vi "ActionVIOnCompile.vi"(8 "error in":errorcluster, 11 "Device Item Ref in":T1 format="%.0x") -> (0 "error out":errorcluster)   [LabVIEW 2017, in "Waveform-Processing-Custom-Device System Explorer.lvlib"]
uses:
  Waveform-Processing-Custom-Device System Explorer.lvlib
  <vilib>/NI Veristand/Custom Device API/Custom Device Item Ref.ctl
  Shared/Types/FG Action.ctl
  Shared/CompiledSettings.ctl
  <vilib>/NI Veristand/Custom Device API/Block Data Reference.ctl
  <vilib>/NI Veristand/Custom Device API/Data Reference.ctl
  <vilib>/NI Veristand/Custom Device API/Waveform Data Reference.ctl
  Shared/Constants.vi
  <vilib>/NI Veristand/Custom Device API/Set Item Property (Variant).vi
  <vilib>/NI Veristand/Custom Device API/Custom Device API.lvlib
  <vilib>/NI/NIVS Inline Async API/_Data Access System Explorer/Data Access System Explorer.lvlib
  Shared/Waveform-Processing-Custom-Device Shared.lvlib
  Shared/Running Average/Running Average.lvlib
  Shared/Single Point/SinglePoint.lvlib
  Shared/Max Single Point/Max_SP.lvlib
  Shared/Min Single Point/Min_SP.lvlib
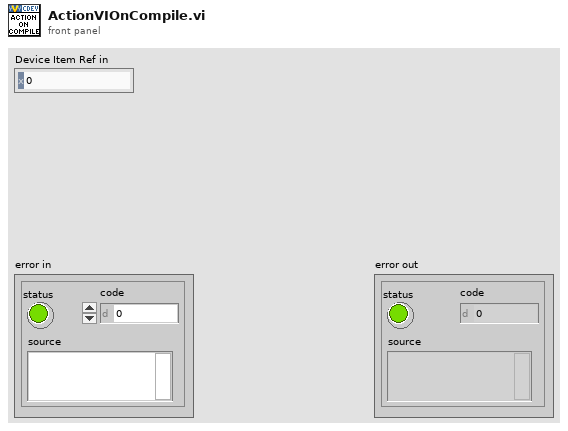
[diagram p1: front panel]
types:
  T1 = typedef "Custom Device API.lvlib/Custom Device Item Ref.ctl" = u64
  T2 = typedef "Waveform-Processing-Custom-Device Shared.lvlib/CompiledSettings.ctl" = cluster{"Name":string, "Buffer Length (samples)":u32, "Enable Array":bool[], "Parameter Block Data Refs":T3[], "Source Wfm Data Refs":T5[], "Result Wfm Data Refs":T5[], "Result Ch Data Refs":T4[], "Task Rate (Hz)":dbl}
  T3 = typedef "Custom Device API.lvlib/Block Data Reference.ctl" = cluster{"Data Reference":T4, "Offset":u64, "Length":u64}
  T4 = typedef "Custom Device API.lvlib/Data Reference.ctl" = i32
  T5 = typedef "Custom Device API.lvlib/Waveform Data Reference.ctl" = i32
  T6 = typedef "Waveform-Processing-Custom-Device Shared.lvlib/FG Action.ctl" = enum8{"GET", "SET"}
  T7 = typedef "Custom Device API.lvlib/Custom Device Item Info.ctl" = cluster{"Name":string, "Is Channel":bool, "GUID":string, "Is Waveform":bool}
  T8 = typedef "Waveform-Processing-Custom-Device Shared.lvlib/Custom Device Settings.ctl" = cluster{"CD Task Dependency":T1, "CD Task Dependency Ref":T1, "CD Task Available Wfms":string[], "CD Task Selected Wfms":string[], "Buffer Length (samples)":u32, "Min Enabled":bool, "Max Enabled ":bool, "SP Enabled":bool, "RMS Enabled":bool, "Buffer Length (s)":dbl, "Task Rate":dbl, "Number of DAQ Chanels":u32}
  T9 = cluster{"Name":string, "Type":enum16{"Output/Write", "Input/Read", "Input/ReadWrite"}, "VS Refs":T1[]}[]
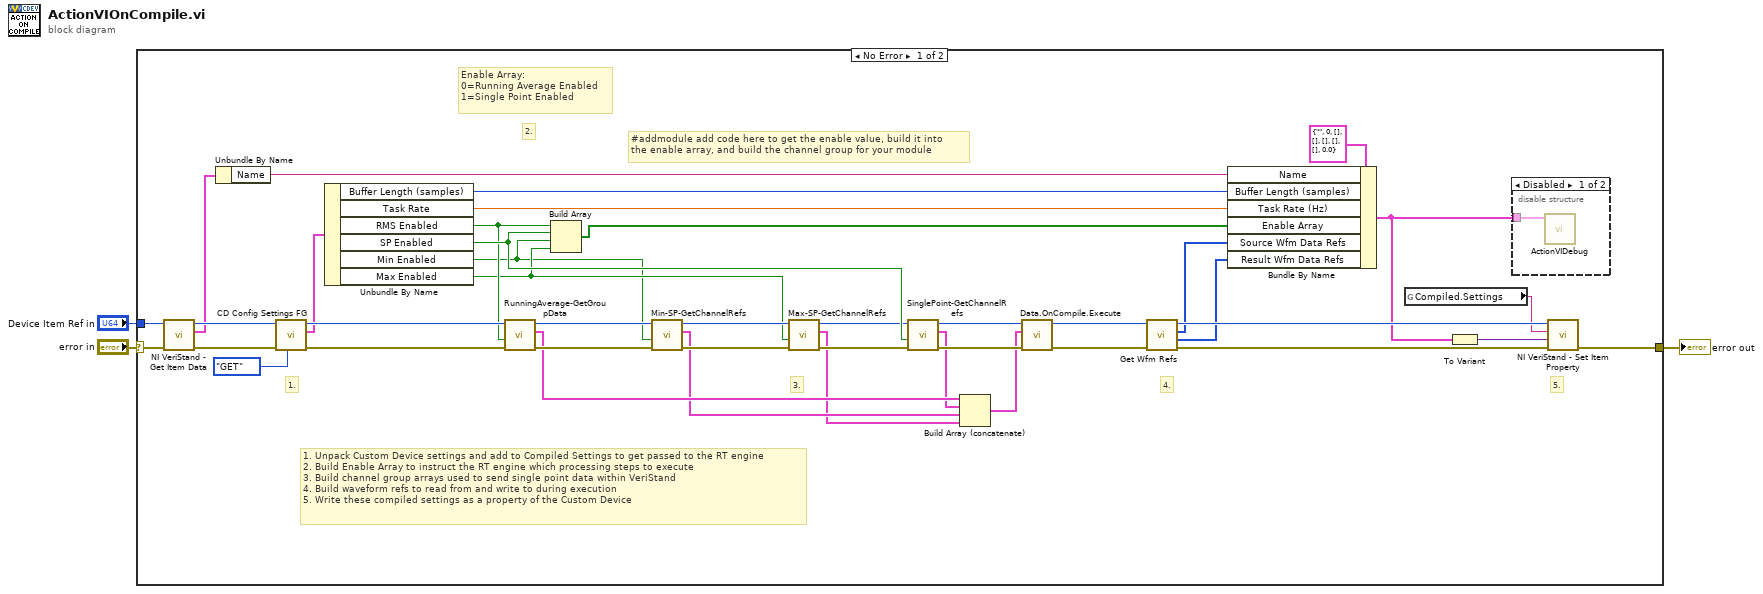
[diagram p0: block diagram]
diagram:
  n1 = case shown="No Error" "error in" {
    selector: "error in" -> [w43 w46]
    tunnel: [w44 w46] -> w2
    tunnel: "Device Item Ref in" -> [w42 _]
    frame No Error {
      # "#addmodule add code here to get the enable value, build it into\nthe enable array, and build the channel group for your module"
      # "Enable Array:\n0=Running Average Enabled\n1=Single Point Enabled"
      # "5."
      # "4."
      # "3."
      # "2."
      # "1."
      # "1. Unpack Custom Device settings and add to Compiled Settings to get passed to the RT engine\n2. Build Enable Array to instruct the RT engine which processing steps to execute\n3. Build channel group arrays used to send single point data within VeriStand\n4. Build waveform refs to read from and write to during execution\n5. Write these compiled settings as a property of the Custom Device"
      n2 = call <vilib>:"NI VeriStand - Get Item Data.vi"("error in (no error)"=w43, "Item Ref in"=w42) -> ("error out"=w40:errorcluster, "Item Info"=w39:T7, "Item Ref out"=w41:T1)  [unwired: 6 in, 1 out]
      n3 = Unbundle By Name(w39) -> ("Name"=w31:string)
      n4 = call "CD Config Settings FG.vi"("Action"=FG_Action."GET", "Error In"=w40, "Item Ref"=w41) -> ("Error Out"=w37:errorcluster, "CD Settings out"=w30:T8, "Item Ref out"=w33:T1)  [unwired: 5 in, 1 out]
      n5 = Unbundle By Name(w30) -> ("Buffer Length (samples)"=w29:u32, "Task Rate"=w20:dbl, "RMS Enabled"=w22:bool, "SP Enabled"=w23:bool, "Min Enabled"=w8:bool, "Max Enabled"=w10:bool)
      n6 = call "RunningAverage-GetGroupData.vi"("Error in"=w37, "Enabled?"=w22, "Device Ref in"=w33) -> ("Error out"=w15:errorcluster, "Group Data Array"=w7:T9, "Device Ref out"=w9:T1)  [unwired: 6 in]
      n7 = Build Array(w22, w23, w8, w10) -> (w21:bool[])
      n8 = call "Min-SP-GetChannelRefs.vi"("Error In"=w15, "OK Button"=w8, "Device Ref in"=w9) -> ("Error Out"=w14:errorcluster, "Group Data Array"=w5:T9, "Device Ref out"=w11:T1)  [unwired: 6 in]
      n9 = call "Max-SP-GetChannelRefs.vi"("Error In"=w14, "Enabled?"=w10, "Device Ref in"=w11) -> ("Error Out"=w13:errorcluster, "Group Data Array"=w4:T9, "Device Ref out"=w12:T1)  [unwired: 6 in]
      n10 = call "SinglePoint-GetChannelRefs.vi"("Error in"=w13, "Enabled?"=w23, "Device Ref in"=w12) -> ("Error out"=w26:errorcluster, "Group Data Array"=w6:T9, "Device Ref out"=w28:T1)  [unwired: 6 in]
      n11 = Build Array (concatenate)(w7, w6, w5, w4) -> (w24:T9)
      n12 = call <vilib>:"Data.OnCompile.Execute.vi"("error in"=w26, "VS Ref Groups"=w24, "Custom Device Ref"=w28) -> ("error out"=w25:errorcluster, "Custom Device Ref"=w27:T1)  [unwired: 7 in]
      n13 = call "Get Wfm Refs.vi"("Error in"=w25, "Device Ref in"=w27) -> ("Error out"=w36:errorcluster, "Results Wfm Data Refs"=w18:T5[], "Source Wfm Data Refs"=w19:T5[], "Device Ref out"=w32:T1)  [unwired: 6 in]
      n14 = Bundle By Name(cluster=T2 {"Name"="", "Buffer Length (samples)"=0, "Enable Array"=[], "Parameter Block Data Refs"=[], "Source Wfm Data Refs"=[], "Result Wfm Data Refs"=[], "Result Ch Data Refs"=[], "Task Rate (Hz)"=0.0} ("CompiledSettings"), "Name"=w31, "Buffer Length (samples)"=w29, "Task Rate (Hz)"=w20, "Enable Array"=w21, "Source Wfm Data Refs"=w19, "Result Wfm Data Refs"=w18) -> (w16:T2)
      n15 = global read "Constants.vi" "Compiled.Settings"() -> (w17:string)
      n16 = To Variant(anything=w16) -> (Variant=w34:variant)
      n17 = disable-structure shown="Disabled" {
        disable-tunnel: w16 -> [w45 _]
        frame Disabled {
          n18 = call "ActionVIDebug.vi"("CompiledSettings"=w45) -> ()  [unwired: 11 in]
        }
        frame Enabled {
        }
      }
      n19 = call-poly <vilib>:"NI VeriStand - Set Item Property.vi"("error in (no error)"=w36, "Value"=w34, "Property Name"=w17, "Item Ref in"=w32) -> ("error out"=w44:errorcluster)  [unwired: 5 in, 2 out]
    }
    frame Error {
    }
  }
  "error out" <- w2
